vi "2DHisto.vi"(9 "Array 2":i32[](array[numeric]), 10 "Array 4":i32[](array[numeric]), 11 "Array":i32[][](array[numeric])) -> (3 "Array 3":i32[][](array[numeric]))   [LabVIEW 2017]
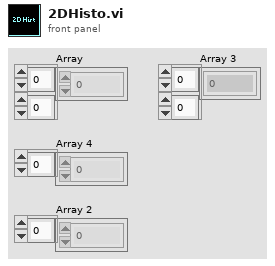
[diagram p1: front panel]
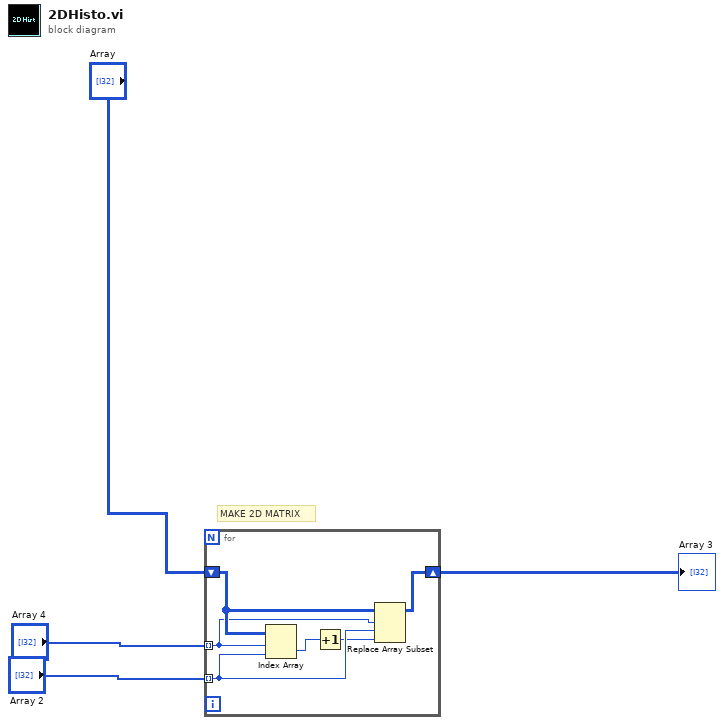
[diagram p0: block diagram]
diagram:
  # "MAKE 2D MATRIX"
  n1 = for {
    shift-right: [w10] -> w2
    shift-left: "Array" -> [w9]
    tunnel: "Array 4" -> [w8] mode=indexing
    tunnel: "Array 2" -> [w7] mode=indexing
    n2 = Index Array(array=w9, index (row)=w8, index (col)=w7) -> (element=w6:i32)
    n3 = Increment(x=w6) -> (x+1=w5:i32)
    n4 = Replace Array Subset(array=w9, new element=w5, index (row)=w8, index (col)=w7) -> (w10:i32[][])
  }
  "Array 3" <- w2
